vi "Fdx Wait for Good Link.vi"(6 "retry period (ms)":u32=200, 8 "error in":errorcluster, 9 "timeout (ms)":u32=10000, 10 "port id":i32=-1, 11 "InstrumentHandle_board in":u32) -> (0 "error out":errorcluster, 1 "timed out":bool, 2 "good link":bool, 3 "InstrumentHandle_board out":u32)   [LabVIEW 2020, in "AIM664LV.lvlib"]
doc: "Waits the amount of time specified in timeout (ms) for the link to the port to FDX_GOOD_LINK. If the port id is not specified, the function will wait for all ports in the board to be FDX_GOOD_LINK. The function uses retry period (ms) to try again. If the board doesn't provide a FDX_GOOD_LINK, then it will return an error."
uses:
  AIM664LV.lvlib
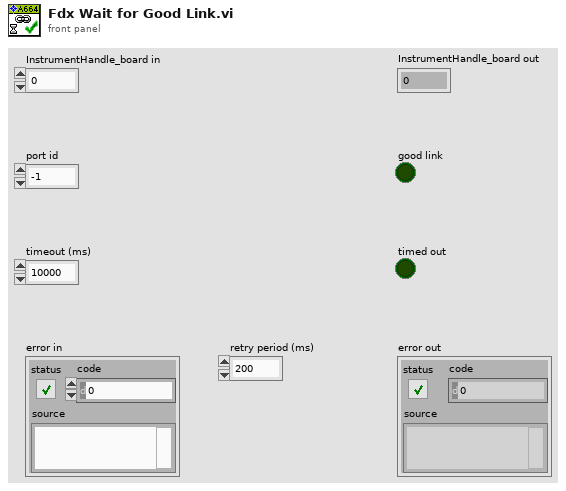
[diagram p1: front panel]
types:
  T1 = typedef "AIM664LV.lvlib/port_configuration.ctl" = u32
  T2 = typedef "AIM664LV.lvlib/port_speed.ctl" = u32
  T3 = typedef "AIM664LV.lvlib/port_condition.ctl" = u32
  T4 = typedef "AIM664LV.lvlib/expert_mode.ctl" = u32
  T5 = cluster{"PortConfig":T1[], "PortSpeed":T2[], "PortUsed":u32[], "PortGoodLink":T3[], "ExpertMode":T4[], "GlobalMemFree":u32, "SharedMemFree":u32, "RxVeriMode":u32}
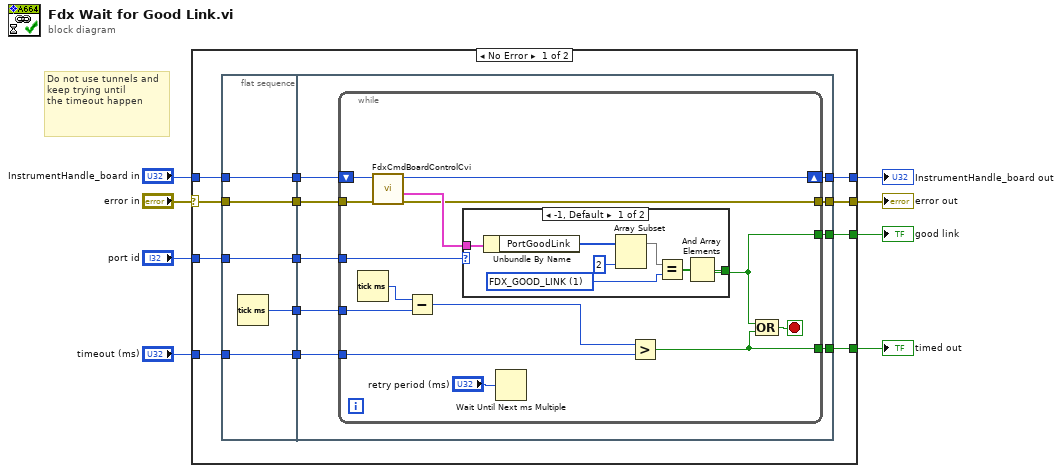
[diagram p0: block diagram]
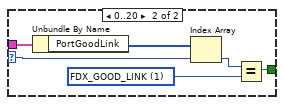
[diagram p2: hidden frame]
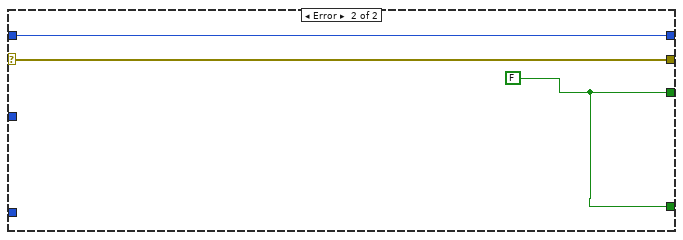
[diagram p3: hidden frame]
diagram:
  # "Do not use tunnels and keep trying until\nthe timeout happen"
  n1 = case shown="No Error" "error in" {
    selector: "error in" -> [w16 w65]
    tunnel: "timeout (ms)" -> [w21 _]
    tunnel: "port id" -> [w20 _]
    tunnel: [w19 w64] -> w5
    tunnel: [w18 w64] -> w6
    tunnel: [w17 w65] -> w7
    tunnel: "InstrumentHandle_board in" -> [w15 w63]
    tunnel: [w9 w63] -> w1
    frame No Error {
      n2 = flat-sequence {
        tunnel: w15 -> [w23]
        tunnel: w16 -> [w24]
        tunnel: w20 -> [w25]
        tunnel: w21 -> [w26]
        tunnel: [w26] -> w14
        tunnel: [w25] -> w13
        tunnel: [w24] -> w12
        tunnel: [w23] -> w11
        tunnel: [w22] -> w10
        tunnel: [w33] -> w19
        tunnel: [w32] -> w18
        tunnel: [w31] -> w17
        tunnel: w14 -> [w35]
        tunnel: w13 -> [w34]
        tunnel: w12 -> [w30]
        tunnel: w11 -> [w29]
        tunnel: w10 -> [w28]
        tunnel: [w27] -> w9
        frame #0 {
          n3 = Tick Count (ms)() -> (millisecond timer value=w22:u32)
        }
        frame #1 {
          n4 = while {
            tunnel: w35 -> [w48]
            tunnel: w34 -> [w36]
            tunnel: [w43] -> w33
            tunnel: [w42] -> w32
            tunnel: w28 -> [w39]
            shift-right: [w38] -> w27
            shift-left: w29 -> [w40]
            tunnel: w30 -> [w41]
            tunnel: [w37] -> w31
            stop <- w44 stop-if-true
            n5 = Tick Count (ms)() -> (millisecond timer value=w47:u32)
            n6 = call "FdxCmdBoardControlCvi.vi"("error in"=w41, "InstrumentHandle_board in"=w40) -> ("error out"=w37:errorcluster, "Board Control Out"=w49:T5, "InstrumentHandle_board out"=w38:u32)  [unwired: 7 in]
            n7 = Subtract(x=w47, y=w39) -> (x-y=w45:u32)
            n8 = case shown="-1, Default" w36 {
              selector: w36 -> [_ w57]
              tunnel: w49 -> [w56 w62]
              tunnel: [w52 w58] -> w42
              frame -1, Default {
                w55 = u32 1 items=["FDX_NO_LINK", "FDX_GOOD_LINK"]
                n9 = Unbundle By Name(w56) -> ("PortGoodLink"=w54:T3[])
                n10 = Array Subset(array=w54, length=2) -> (w51:T3[])  [unwired: 1 in]
                n11 = Equal?(x=w51, y=w55) -> (x = y?=w53:bool[])
                n12 = And Array Elements(Boolean array=w53) -> (logical AND=w52:bool)
              }
              frame 0..20 {
                w59 = u32 1 items=["FDX_NO_LINK", "FDX_GOOD_LINK"]
                n13 = Unbundle By Name(w62) -> ("PortGoodLink"=w61:T3[])
                n14 = Index Array(array=w61, index=w57) -> (element=w60:T3)
                n15 = Equal?(x=w60, y=w59) -> (x = y?=w58:bool)
              }
            }
            n16 = Wait Until Next ms Multiple(millisecond multiple="retry period (ms)") -> ()  [unwired: 1 out]
            n17 = Greater?(x=w45, y=w48) -> (0:w43:bool)
            n18 = Compound Arithmetic op=OR(w42, w43) -> (w44:bool)
          }
        }
      }
    }
    frame Error {
      w64 = FALSE
    }
  }
  "error out" <- w7
  "good link" <- w6
  "timed out" <- w5
  "InstrumentHandle_board out" <- w1
